vi "지진계측기(교수님 코드)_AI 및 DI 추가 스위치 제어_생성자 소비자.vi"() -> ()   [LabVIEW 2020]
uses:
  <vilib>/DAQmx/read.llb/DAQmx Read (Analog 1D DBL 1Chan NSamp).vi
  <vilib>/Analysis/baseanly.llb/Mean (DBL).vi
  <vilib>/DAQmx/read.llb/DAQmx Read (Digital U8 1Chan 1Samp).vi
  <vilib>/DAQmx/create/channels.llb/DAQmx Create Channel (DI-Digital Input).vi
  <vilib>/DAQmx/miscellaneous.llb/DAQmx Fill In Error Info.vi
  <vilib>/DAQmx/create/channels.llb/DAQmx Create Channel (AI-Voltage-Basic).vi
  <vilib>/DAQmx/configure/timing.llb/DAQmx Timing (Sample Clock).vi
  <vilib>/Analysis/NI_AALBase.lvlib
panel:
  out "문자열":string
  out "알람발생":bool
  out "웨이브폼 차트":dbl(graph)
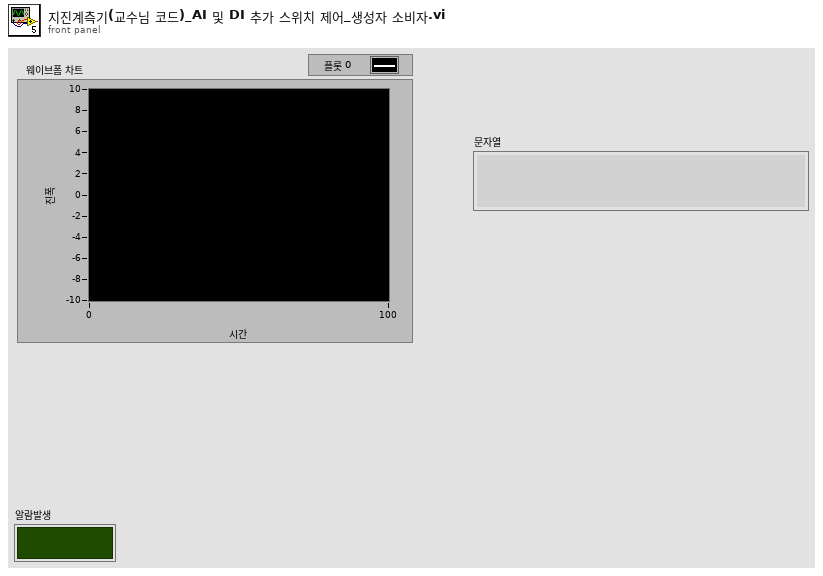
[diagram p1: front panel]
types:
  T1 = enum16{"초기화", "감지 시작", "지진감지", "알람 발생", "알람 리셋", "정지"}
  T2 = cluster{"DI Task":refnum<k21>, "DI Q":refnum<queue>, "중복":bool}
  T3 = cluster{"AI":refnum<k21>, "알람 발생":bool, "데이터":dbl, "알람 데이터":string}
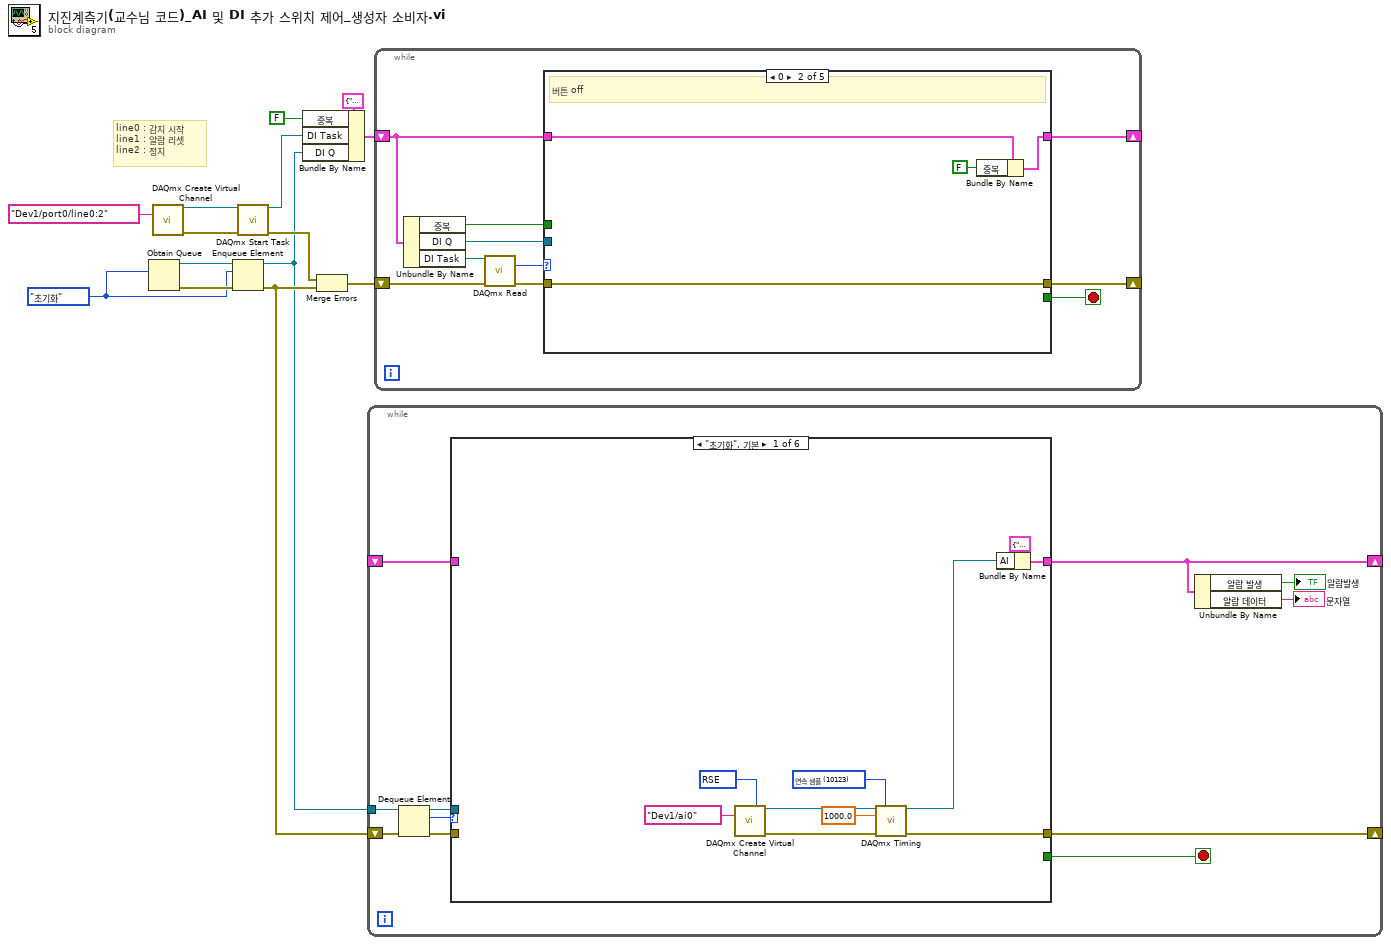
[diagram p0: block diagram]
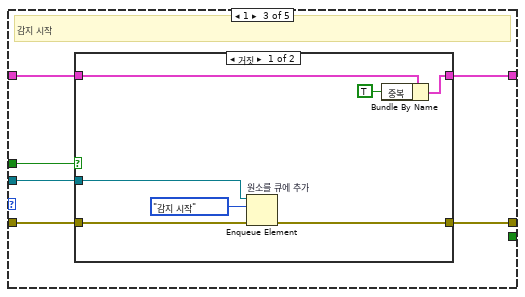
[diagram p3: hidden frame]
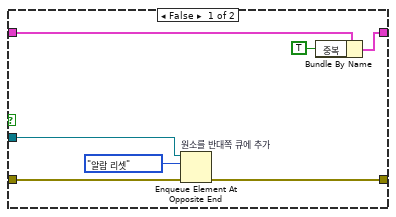
[diagram p6: hidden frame]
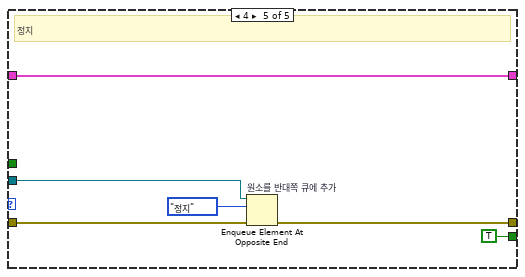
[diagram p7: hidden frame]
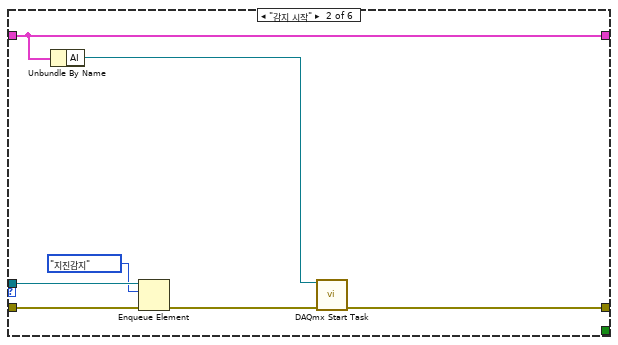
[diagram p8: hidden frame]
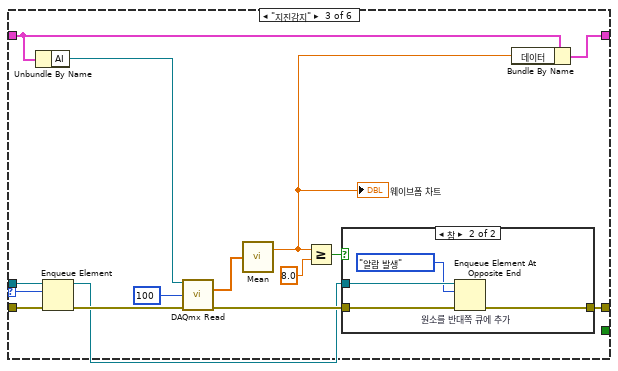
[diagram p9: hidden frame]
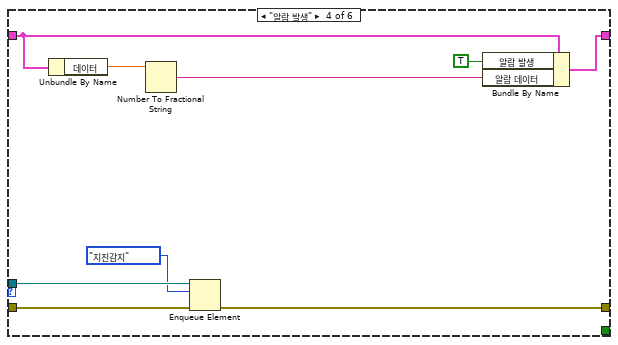
[diagram p11: hidden frame]
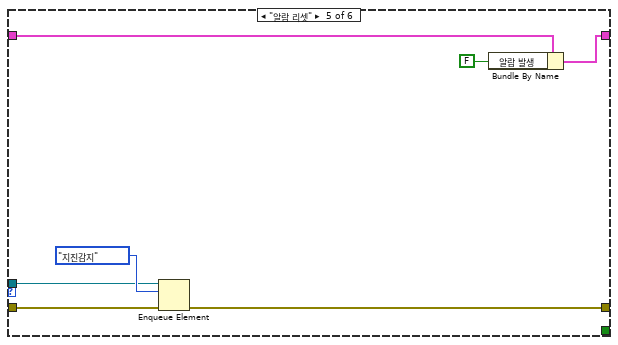
[diagram p12: hidden frame]
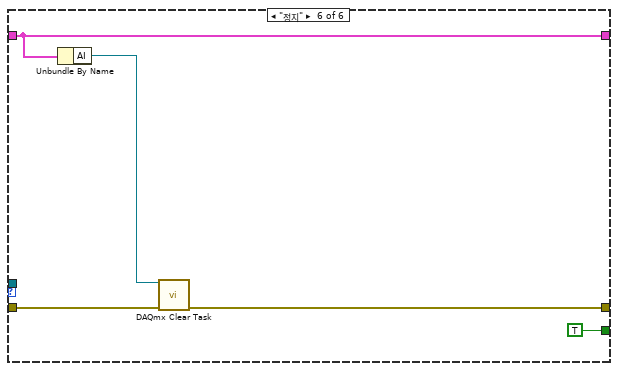
[diagram p13: hidden frame]
diagram:
  w5 = T1."초기화"
  # "line0 : 감지 시작\nline1 : 알람 리셋\nline2 : 정지"
  n1 = Obtain Queue(element data type=w5) -> (queue out=w7:refnum<queue>, error out=w6:errorcluster)  [unwired: 4 in, 1 out]
  n2 = call-poly <vilib>:"DAQmx Create Virtual Channel.vi"("lines"=tag "Dev1/port0/line0:2") -> ("task out"=w13:refnum<k21>, "error out"=w12:errorcluster)  [unwired: 13 in]
  n3 = Enqueue Element(queue=w7, element=w5, error in (no error)=w6) -> (queue out=w1:refnum<queue>, error out=w2:errorcluster)  [unwired: 1 in, 1 out]
  n4 = call <vilib>:"DAQmx Start Task.vi"("task/channels in"=w13, "error in"=w12) -> ("task out"=w10:refnum<k21>, "error out"=w4:errorcluster)  [unwired: 12 in]
  n5 = Bundle By Name(cluster=T2 {"DI Task"="", "DI Q"=refnum, "중복"=FALSE}, "중복"=FALSE, "DI Task"=w10, "DI Q"=w1) -> (w8:T2)
  n6 = Merge Errors(w4, w2) -> (w3:errorcluster)
  n7 = while {
    shift-right: [w24] -> _
    shift-left: _ -> [w25]
    shift-right: [w20] -> _
    shift-left: w2 -> [w19]
    tunnel: w1 -> [w18]
    stop <- w22 stop-if-true
    n8 = Dequeue Element(queue=w18, error in (no error)=w19) -> (queue out=w15:refnum<queue>, element=w17:T1, error out=w16:errorcluster)  [unwired: 1 in, 1 out]
    n9 = case shown="\"초기화\", 기본" w17 {
      selector: w17 -> [_ _ w45 _ _ _]
      tunnel: [w28 w42 w54 w71 w77 w82] -> w24
      tunnel: w25 -> [_ w42 w51 w69 w78 w82]
      tunnel: w16 -> [_ w39 w47 w66 w74 w80]
      tunnel: [w26 w40 w48 w63 w72 w79] -> w20
      tunnel: [_ _ _ _ _ TRUE] -> w22
      tunnel: w15 -> [_ w38 w46 w65 w73 _]
      frame "초기화", Default {
        w31 = 10123 items=["유한 샘플"=10178, "연속 샘플"=10123, "하드웨어 타이밍에 의한 단일 포인트"=12522] ("sample mode")
        w32 = 10083 items=["기본"=-1, "RSE"=10083, "NRSE"=10078, "차동"=10106, "유사 차동"=12529] ("input terminal configuration")
        n10 = call-poly <vilib>:"DAQmx Create Virtual Channel.vi"("input terminal configuration"=w32, "physical channels"=tag "Dev1/ai0") -> ("task out"=w35:refnum<k21>, "error out"=w34:errorcluster)  [unwired: 12 in]
        n11 = call-poly <vilib>:"DAQmx Timing.vi"("task/channels in"=w35, "sample mode"=w31, "rate"=1000.0, "error in"=w34) -> ("task out"=w27:refnum<k21>, "error out"=w26:errorcluster)  [unwired: 10 in]
        n12 = Bundle By Name(cluster=T3 {"AI"="", "알람 발생"=FALSE, "데이터"=0.0, "알람 데이터"=""}, "AI"=w27) -> (w28:T3)
      }
      frame "감지 시작" {
        n13 = Unbundle By Name(w42) -> ("AI"=w41:refnum<k21>)
        n14 = Enqueue Element(queue=w38, element=T1."지진감지" ("원소"), error in (no error)=w39) -> (error out=w37:errorcluster)  [unwired: 1 in, 2 out]
        n15 = call <vilib>:"DAQmx Start Task.vi"("task/channels in"=w41, "error in"=w37) -> ("error out"=w40:errorcluster)  [unwired: 12 in, 1 out]
      }
      frame "지진감지" {
        n16 = Unbundle By Name(w51) -> ("AI"=w52:refnum<k21>)
        n17 = Enqueue Element(queue=w46, element=w45, error in (no error)=w47) -> (queue out=w43:refnum<queue>, error out=w44:errorcluster)  [unwired: 1 in, 1 out]
        n18 = call-poly <vilib>:"DAQmx Read.vi"("task/channels in"=w52, "number of samples per channel"=100, "error in"=w44) -> ("data"=w56:dbl[], "error out"=w50:errorcluster)  [unwired: 10 in, 1 out]
        n19 = call-poly <vilib>:"Mean.vi"("X"=w56) -> ("mean"=w53:dbl)  [unwired: 1 out]
        "웨이브폼 차트" <- w53
        n20 = Greater Or Equal?(x=w53, y=8.0) -> (x >= y?=w49:bool)
        n21 = case shown="참" w49 {
          tunnel: w50 -> [w58 w62]
          tunnel: w43 -> [_ w61]
          tunnel: [w58 w59] -> w48
          frame False {
          }
          frame True {
            n22 = Enqueue Element At Opposite End "원소를 반대쪽 큐에 추가"(queue=w61, element=T1."알람 발생" ("원소"), error in (no error)=w62) -> (error out=w59:errorcluster)  [unwired: 1 in, 2 out]
          }
        }
        n23 = Bundle By Name(cluster=w51, "데이터"=w53) -> (w54:T3)
      }
      frame "알람 발생" {
        n24 = Unbundle By Name(w69) -> ("데이터"=w68:dbl)
        n25 = Number To Fractional String(number=w68) -> (F-format string=w67:string)  [unwired: 3 in]
        n26 = Enqueue Element(queue=w65, element=T1."지진감지" ("원소"), error in (no error)=w66) -> (error out=w63:errorcluster)  [unwired: 1 in, 2 out]
        n27 = Bundle By Name(cluster=w69, "알람 발생"=TRUE, "알람 데이터"=w67) -> (w71:T3)
      }
      frame "알람 리셋" {
        n28 = Enqueue Element(queue=w73, element=T1."지진감지" ("원소"), error in (no error)=w74) -> (error out=w72:errorcluster)  [unwired: 1 in, 2 out]
        n29 = Bundle By Name(cluster=w78, "알람 발생"=FALSE) -> (w77:T3)
      }
      frame "정지" {
        n30 = Unbundle By Name(w82) -> ("AI"=w81:refnum<k21>)
        n31 = call <vilib>:"DAQmx Clear Task.vi"("task in"=w81, "error in"=w80) -> ("error out"=w79:errorcluster)  [unwired: 13 in]
      }
    }
    n32 = Unbundle By Name(w24) -> ("알람 발생"=→"알람발생":bool, "알람 데이터"=→"문자열":string)
  }
  n33 = while {
    shift-right: [w86] -> _
    shift-left: w8 -> [w87]
    shift-right: [w88] -> _
    shift-left: w3 -> [w93]
    stop <- w84 stop-if-true
    n34 = Unbundle By Name(w87) -> ("중복"=w90:bool, "DI Q"=w85:refnum<queue>, "DI Task"=w91:refnum<k21>)
    n35 = call-poly <vilib>:"DAQmx Read.vi"("task/channels in"=w91, "error in"=w93) -> ("data"=w92:u8, "error out"=w89:errorcluster)  [unwired: 11 in, 1 out]
    n36 = case shown="0" w92 {
      tunnel: w90 -> [_ _ w105 w120 _]
      tunnel: w89 -> [w94 w96 w102 w117 w135]
      tunnel: [w94 w96 w101 w116 w134] -> w88
      tunnel: w87 -> [w95 w99 w104 w119 w132]
      tunnel: [w95 w97 w103 w118 w132] -> w86
      tunnel: w85 -> [_ _ w100 w115 w133]
      tunnel: [_ _ _ _ TRUE] -> w84
      frame Default {
        # "버튼 동시 입력"
      }
      frame 0 {
        # "버튼 off"
        n37 = Bundle By Name(cluster=w99, "중복"=FALSE) -> (w97:T2)
      }
      frame 1 {
        # "감지 시작"
        n38 = case shown="거짓" w105 {
          tunnel: w104 -> [w112 w114]
          tunnel: [w111 w114] -> w103
          tunnel: w102 -> [w109 w113]
          tunnel: [w107 w113] -> w101
          tunnel: w100 -> [w108 _]
          frame False {
            n39 = Enqueue Element "원소를 큐에 추가"(queue=w108, element=T1."감지 시작", error in (no error)=w109) -> (error out=w107:errorcluster)  [unwired: 1 in, 2 out]
            n40 = Bundle By Name(cluster=w112, "중복"=TRUE) -> (w111:T2)
          }
          frame True {
          }
        }
      }
      frame 2 {
        # "알람 리셋"
        n41 = case shown="참" w120 {
          tunnel: w119 -> [w127 w129]
          tunnel: [w126 w129] -> w118
          tunnel: w117 -> [w124 w128]
          tunnel: [w122 w128] -> w116
          tunnel: w115 -> [w123 _]
          frame False {
            n42 = Enqueue Element At Opposite End "원소를 반대쪽 큐에 추가"(queue=w123, element=T1."알람 리셋", error in (no error)=w124) -> (error out=w122:errorcluster)  [unwired: 1 in, 2 out]
            n43 = Bundle By Name(cluster=w127, "중복"=TRUE) -> (w126:T2)
          }
          frame True {
          }
        }
      }
      frame 4 {
        # "정지"
        n44 = Enqueue Element At Opposite End "원소를 반대쪽 큐에 추가"(queue=w133, element=T1."정지", error in (no error)=w135) -> (error out=w134:errorcluster)  [unwired: 1 in, 2 out]
      }
    }
  }
